vi "Populate Elements From Document.vi"(8 "error in (no error)":errorcluster, 11 "xwpfDocument in":refnum<class "xwpfDocument.lvclass">) -> (0 "error out":errorcluster, 3 "xwpfDocument out":refnum<class "xwpfDocument.lvclass">)   [LabVIEW 2017, in "Word_Specific.lvlib" / "xwpfDocument.lvclass"]
uses:
  xwpfDocument.lvclass
  xwpfDocument.lvclass/xwpfDocument.ctl
  C:/Users/Neo/Desktop/Dev_Tools_BR/LabVIEW_NPOI/lib/NPOI 2.1.1/NPOI.OOXML.dll
  lib/NPOI 2.1.1/NPOI.OOXML.dll
  xwpfParagraph/xwpfParagraph.lvclass
  C:/Users/Neo/Desktop/Dev_Tools_BR/LabVIEW_NPOI/src/LabVIEW NPOI/xwpfDocument.Element/xwpfDocument.Element.lvclass
  xwpfTable/xwpfTable.lvclass
  xwpfDocument.Element/xwpfDocument.Element.lvclass
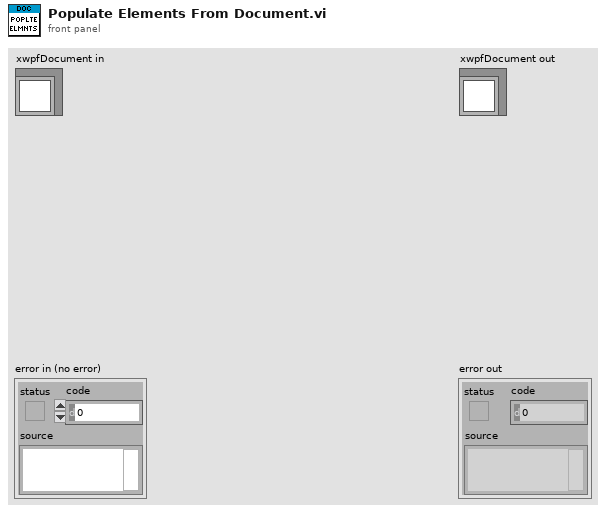
[diagram p1: front panel]
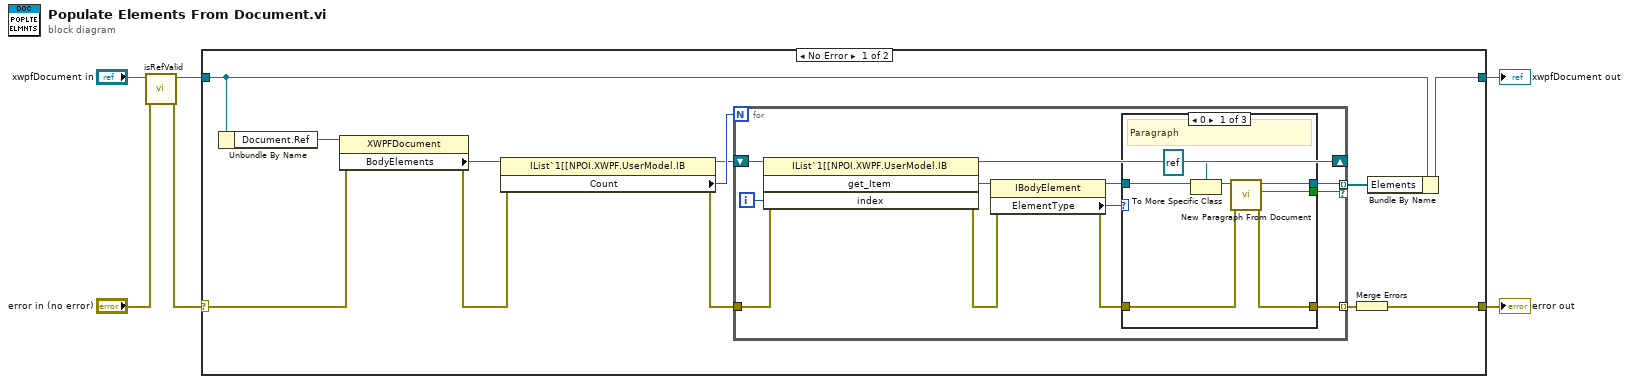
[diagram p0: block diagram]
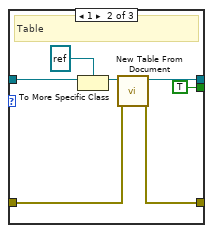
[diagram p2: hidden frame]
diagram:
  n1 = call-dynamic "isRefValid.vi"("error in (no error)"="error in (no error)", "xwpfDocument in"="xwpfDocument in") -> ("error out"=w1:errorcluster, "xwpfDocument out"=w3:refnum<class "xwpfDocument.lvclass">)  [unwired: 8 in]
  n2 = case shown="No Error" w1 {
    selector: w1 -> [w14 w47]
    tunnel: [w11 w47] -> w6
    tunnel: [w8 w46] -> w4
    tunnel: w3 -> [w9 w46]
    frame No Error {
      n3 = Unbundle By Name(w9) -> ("Document.Ref"=w12:refnum<k24>)
      n4 = property class="XWPFDocument"(reference=w12, error in=w14) -> (error out=w15:errorcluster, "BodyElements"=w18:refnum<k24>)  [unwired: 1 out]
      n5 = property class="IList`1[[NPOI.XWPF.UserModel.IB"(reference=w18, error in=w15) -> (reference out=w10:refnum<k24>, error out=w16:errorcluster, "Count"=w17:i32)
      n6 = for {
        N: w17 -> [_]
        shift-right: [w28] -> _
        shift-left: w10 -> [w30]
        tunnel: w16 -> [w27]
        tunnel: [w24] -> w13 mode=indexing
        tunnel: [w21] -> w7 mode=indexing if=w20
        i -> [w29]
        n7 = invoke class="IList`1[[NPOI.XWPF.UserModel.IB" method="get_Item"(reference=w30, error in=w27, "index"=w29) -> (reference out=w28:refnum<k24>, error out=w23:errorcluster, "get_Item"=w26:refnum<k24>)  [unwired: 1 in, 1 out]
        n8 = property class="IBodyElement"(reference=w26, error in=w23) -> (reference out=w25:refnum<k24>, error out=w22:errorcluster, "ElementType"=w19:i32)
        n9 = case shown="0" w19 {
          tunnel: w25 -> [w37 w44 _]
          tunnel: w22 -> [w32 w40 w45]
          tunnel: [w31 w39 w45] -> w24
          tunnel: [w34 w41 _] -> w21
          tunnel: [w33 TRUE ("New Element Found") _] -> w20
          frame 0 {
            # "Paragraph"
            n10 = To More Specific Class(target class=refnum<k24> refnum, reference=w37) -> (specific class reference=w36:refnum<k24>)  [unwired: 1 in, 1 out]
            n11 = call "New Paragraph From Document.vi"("error in (no error)"=w32, "Paragraph Ref"=w36) -> ("error out"=w31:errorcluster, "New Element Found"=w33:bool, "xwpfParagraph out"=w34:refnum<class "xwpfParagraph.lvclass">)  [unwired: 7 in]
          }
          frame 1 {
            # "Table"
            n12 = To More Specific Class(target class=refnum<k24> refnum, reference=w44) -> (specific class reference=w43:refnum<k24>)  [unwired: 1 in, 1 out]
            n13 = call "New Table From Document.vi"("error in (no error)"=w40, "Table Ref"=w43) -> ("error out"=w39:errorcluster, "xwpfTable out"=w41:refnum<class "xwpfTable.lvclass">)  [unwired: 8 in]
          }
          frame Default {
          }
        }
      }
      n14 = Merge Errors(w13) -> (w11:errorcluster)
      n15 = Bundle By Name(cluster=w9, "Elements"=w7) -> (w8:refnum<class "xwpfDocument.lvclass">)
    }
    frame Error {
    }
  }
  "error out" <- w6
  "xwpfDocument out" <- w4
